vi "Status.vi"(8 "error in (no error)":errorcluster, 10 "return elements? (F)":bool, 11 "Queue in":refnum<class "Queue.lvclass">) -> (0 "error out":errorcluster, 1 "# pending insert":i32, 2 "# pending remove":i32, 3 "Queue out":refnum<class "Queue.lvclass">, 4 "# elements in queue":i32, 5 "Queue name":string, 6 "Element":refnum<class "Data.lvclass">[](array[class]), 7 "Max queue size":i32)   [LabVIEW 2020, in "Data.lvlib" / "Queue.lvclass"]
doc: "Get the queue status."
uses:
  Queue.lvclass
  Data.lvclass
  Queue.lvclass/Queue.ctl
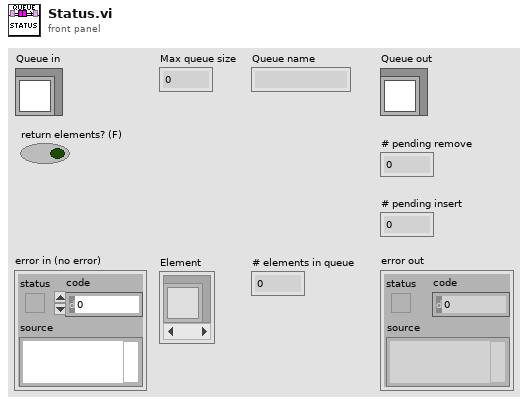
[diagram p1: front panel]
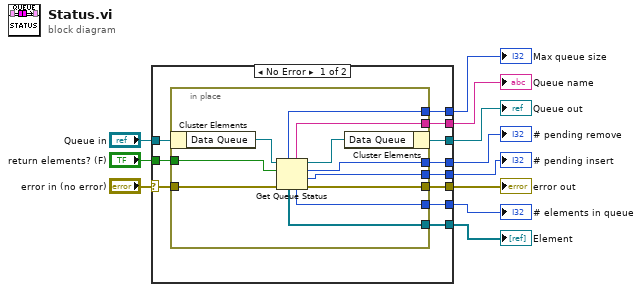
[diagram p0: block diagram]
diagram:
  n1 = case shown="No Error" "error in (no error)" {
    selector: "error in (no error)" -> [w20 w35]
    tunnel: [w19 w35] -> w10
    tunnel: [w21 w34] -> w8
    tunnel: "Queue in" -> [w22 w34]
    tunnel: [w18 _] -> w7
    tunnel: "return elements? (F)" -> [w17 _]
    tunnel: [w16 _] -> w5
    tunnel: [w15 _] -> w4
    tunnel: [w14 _] -> w3
    tunnel: [w13 _] -> w2
    tunnel: [w12 _] -> w1
    frame No Error {
      n2 = in-place {
        in-place-border: w20 -> [w31]
        in-place-border: [w30] -> w19
        in-place-border: [w28] -> w18
        in-place-border: w17 -> [w29]
        in-place-border: [w27] -> w16
        in-place-border: [w26] -> w15
        in-place-border: [w25] -> w14
        in-place-border: [w24] -> w13
        in-place-border: [w23] -> w12
        n3 = in-place-cluster #1(w22) -> ("Data Queue"=w33:refnum<queue>)
        n4 = Get Queue Status(queue=w33, return elements? (F)=w29, error in (no error)=w31) -> (queue out=w32:refnum<queue>, queue name=w26:string, max queue size=w27:i32, # pending remove=w25:i32, # pending insert=w24:i32, error out=w30:errorcluster, # elements in queue=w23:i32, elements=w28:refnum<class "Data.lvclass">[])
        n5 = in-place-cluster #1("Data Queue"=w32) -> (w21:refnum<class "Queue.lvclass">)
      }
    }
    frame Error {
    }
  }
  "error out" <- w10
  "Queue out" <- w8
  "Element" <- w7
  "Max queue size" <- w5
  "Queue name" <- w4
  "# elements in queue" <- w1
  "# pending remove" <- w3
  "# pending insert" <- w2
